vi "MassData Support Prototype.vi"() -> ()   [LabVIEW 2020, in "TCPRouter ClientAPI Examples.lvlib"]
uses:
  <userlib>/_NEVSTOP/Communicable State Machine(CSM)/addons/MassData-Parameter/_support/Operation-FGV-MassData.ctl
  14bf48ef-9347-4052-95a4-096c444b6f5b.vi
  <userlib>/_NEVSTOP/Communicable State Machine(CSM)/Utility/CSM Data Type String.vi
  <userlib>/_NEVSTOP/Communicable State Machine(CSM)/addons/MassData-Parameter/_support/FGV-MassData(lvlibp).vi
  TCPRouter ClientAPI Examples.lvlib
  <userlib>/_NEVSTOP/Communicable State Machine(CSM)/addons/MassData-Parameter/CSM MassData Parameter Support.lvlib
panel:
  out "concatenated string 2":string
  out "concatenated string":string
  out "MassData Argument 2":string
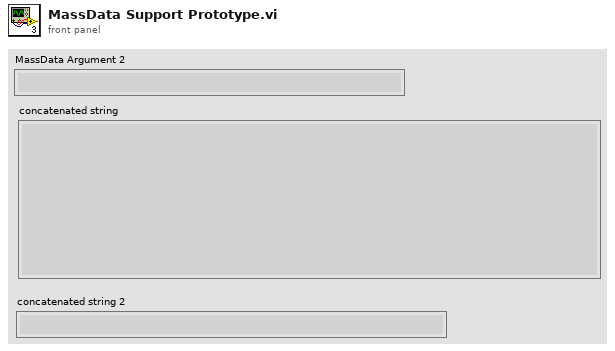
[diagram p1: front panel]
types:
  T1 = typedef "CSM MassData Parameter Support.lvlib/Operation-FGV-MassData.ctl" = enum16{"Initialize", "Read", "Write", "Status", "Release"}
  T2 = typedef "CSM MassData Parameter Support.lvlib/Def-MassDataOper-Status.ctl" = cluster{"Start":i32, "Size":i32, "Total":i32}
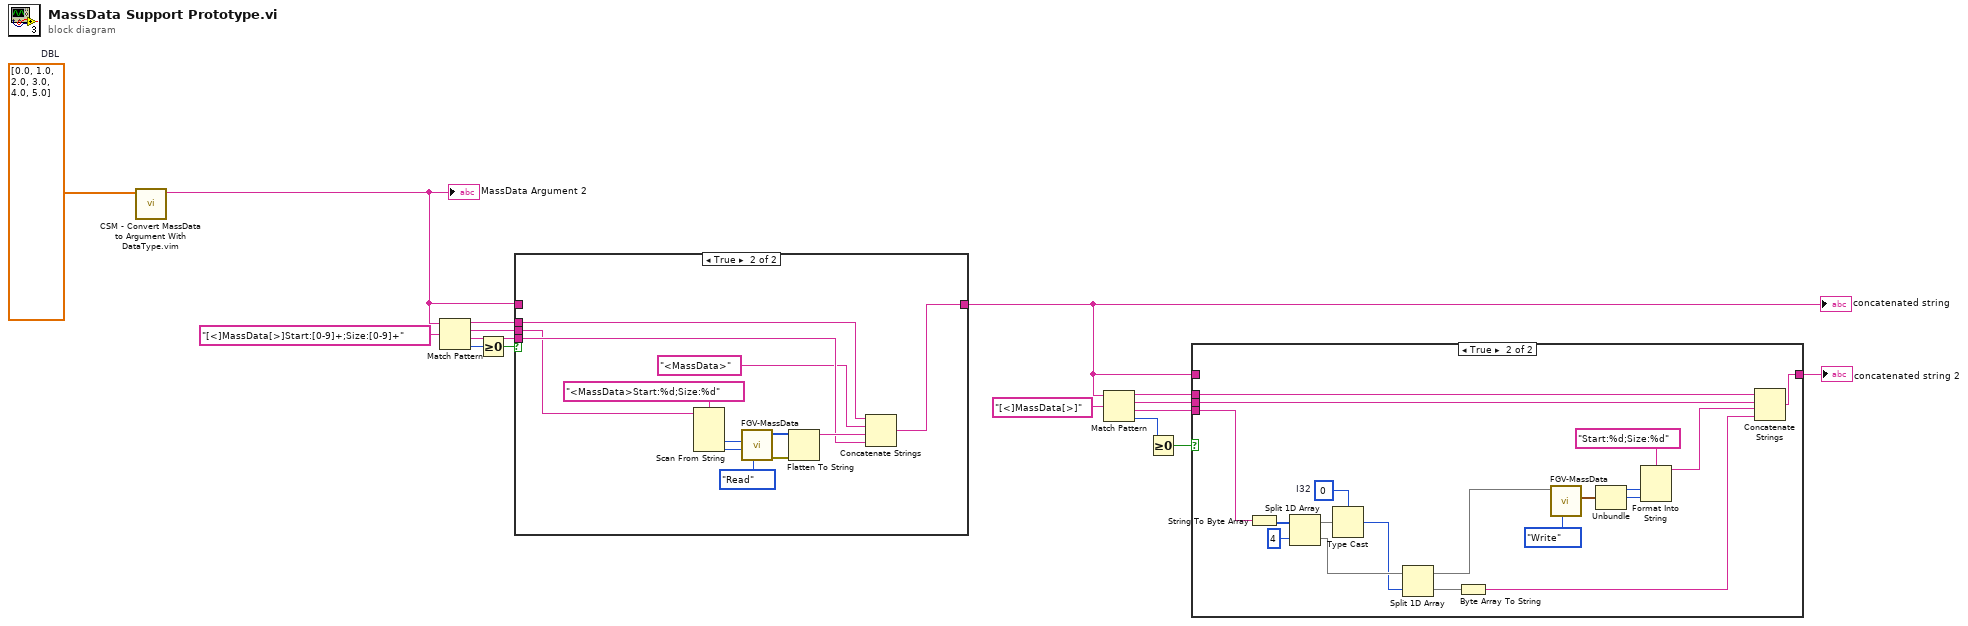
[diagram p0: block diagram]
diagram:
  w16 = dbl[] [0.0, 1.0, 2.0, 3.0, 4.0, 5.0]  # DBL
  n1 = call "CSM - Convert MassData to Argument With DataType.vim"("Data"=w16) -> ("MassData Argument"=w9:string)  [unwired: 7 in, 1 out]
  "MassData Argument 2" <- w9
  n2 = Match Pattern(string=w9, regular expression="[<]MassData[>]Start:[0-9]+;Size:[0-9]+" ("string")) -> (before substring=w14:string, match substring=w12:string, after substring=w13:string, offset past match=w11:i32)  [unwired: 1 in]
  n3 = Greater Or Equal To 0?(x=w11) -> (x >= 0?=w10:bool)
  n4 = case shown="True" w10 {
    tunnel: w14 -> [_ w24]
    tunnel: w13 -> [_ w23]
    tunnel: [w17 w22] -> w1
    tunnel: w12 -> [_ w21]
    tunnel: w9 -> [w17 _]
    frame False {
    }
    frame True {
      n5 = Scan From String(format string="<MassData>Start:%d;Size:%d", input string=w21) -> (output 1=w28:i32, output 2=w27:i32)  [unwired: 4 in, 3 out]
      n6 = call <userlib>:"FGV-MassData.vi"("Operation"=Operation-FGV-MassData."Read", "size"=w27, "Start"=w28) -> ("Error out"=w18:errorcluster, "Data out"=w26:u8[])  [unwired: 5 in, 2 out]
      n7 = Flatten To String(anything=w26, error in (no error)=w18) -> (data string=w25:string)  [unwired: 2 in, 2 out]
      n8 = Concatenate Strings(w24, "<MassData>" ("format string"), w25, w23) -> (w22:string)
    }
  }
  "concatenated string" <- w1
  n9 = Match Pattern(string=w1, regular expression="[<]MassData[>]" ("string")) -> (before substring=w6:string, match substring=w5:string, after substring=w4:string, offset past match=w7:i32)  [unwired: 1 in]
  n10 = Greater Or Equal To 0?(x=w7) -> (x >= 0?=w2:bool)
  n11 = case shown="True" w2 {
    tunnel: w6 -> [_ w49]
    tunnel: w5 -> [_ w48]
    tunnel: w4 -> [_ w47]
    tunnel: [w30 w31] -> w3
    tunnel: w1 -> [w30 _]
    frame False {
    }
    frame True {
      w43 = 0  # I32
      n12 = String To Byte Array(string=w47) -> (unsigned byte array=w46:u8[])
      n13 = Split 1D Array(array=w46, index=4) -> (first subarray=w44:u8[], second subarray=w42:u8[])
      n14 = Type Cast(type=w43, x=w44) -> (*(type *) &x=w41:i32)
      n15 = Split 1D Array(array=w42, index=w41) -> (first subarray=w33:u8[], second subarray=w40:u8[])
      n16 = Byte Array To String(unsigned byte array=w40) -> (string=w39:string)
      n17 = call <userlib>:"FGV-MassData.vi"("Operation"=Operation-FGV-MassData."Write", "Data in"=w33) -> ("Active Write Oper"=w37:T2)  [unwired: 6 in, 3 out]
      n18 = Unbundle(w37) -> ("Start"=w36:i32, "Size"=w35:i32)  [unwired: 1 out]
      n19 = Format Into String(format string="Start:%d;Size:%d", w36, w35) -> (resulting string=w32:string)  [unwired: 2 in, 1 out]
      n20 = Concatenate Strings(w49, w48, w32, w39) -> (w31:string)
    }
  }
  "concatenated string 2" <- w3
